vi "Update Display.vi"(8 "error in (no error)":errorcluster, 11 "Text in":refnum<class "Text.lvclass">) -> (0 "error out":errorcluster, 1 "Right":u8[](array[numeric]), 2 "Left":u8[](array[numeric]), 3 "Text out":refnum<class "Text.lvclass">)   [LabVIEW 2026, in "LED Matrix.lvlib" / "Text.lvclass"]
uses:
  Text.lvclass
  home/pete/dev/labview-car/dev/LED Matrix/Content/Content.lvclass
  Text.lvclass/Text.ctl
  Content/Content.lvclass
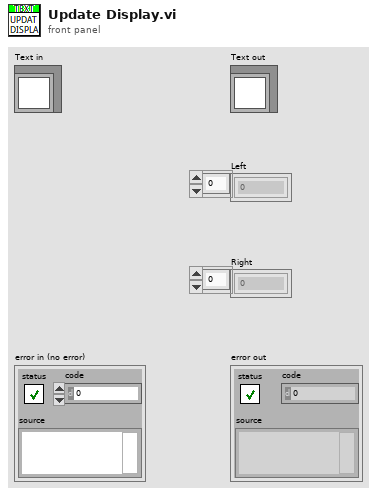
[diagram p1: front panel]
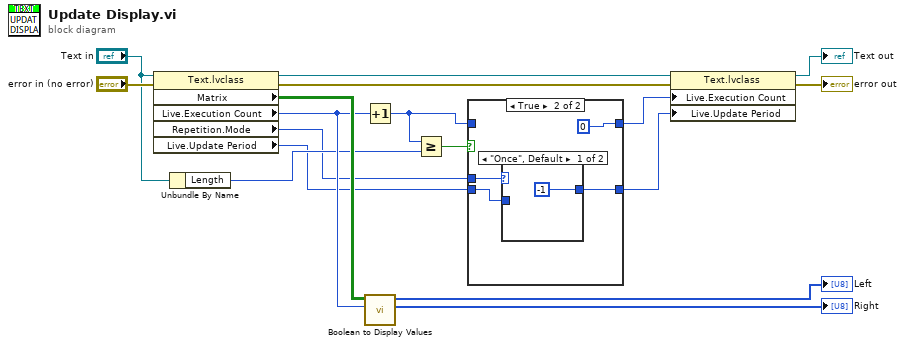
[diagram p0: block diagram]
diagram:
  n1 = property class="Text.lvclass"(reference="Text in", error in="error in (no error)") -> (reference out=w11:refnum<class "Text.lvclass">, error out=w15:errorcluster, "Matrix"=w16:bool[][], "Live.Execution Count"=w9:i32, "Repetition.Mode"=w6:enum16{"Once", "Count", "Infinite"}, "Live.Update Period"=w4:i32)
  n2 = Unbundle By Name("Text in") -> ("Length"=w7:i32)
  n3 = Increment(x=w9) -> (x+1=w2:i32)
  n4 = call "Boolean to Display Values.vi"("Offset"=w9, "Array"=w16) -> ("Right"=→"Right":u8[], "Left"=→"Left":u8[])  [unwired: 8 in]
  n5 = Greater Or Equal?(x=w2, y=w7) -> (x >= y?=w3:bool)
  n6 = case shown="True" w3 {
    tunnel: w6 -> [_ w23]
    tunnel: [w18 w22] -> w5
    tunnel: w4 -> [w18 w21]
    tunnel: w2 -> [w19 _]
    tunnel: [w19 0] -> w1
    frame False {
    }
    frame True {
      n7 = case shown="\"Once\", Default" w23 {
        tunnel: [-1 ("Update Period") w25] -> w22
        tunnel: w21 -> [_ w25]
        frame "Once", Default {
        }
        frame "Infinite" {
        }
      }
    }
  }
  n8 = property class="Text.lvclass"(reference=w11, error in=w15, "Live.Execution Count"=w1, "Live.Update Period"=w5) -> (reference out=→"Text out":refnum<class "Text.lvclass">, error out=→"error out":errorcluster)
